vi "UIM Reg Notice wrapper.vi"(7 "b828NoticeDn":i32[](array[numeric])=[0, 0, 0, 0, 0, 0, 0, 0], 8 "error in (no error)":errorcluster caption="错误输入（无错误）", 9 "b828NoticeUp":i32[](array[numeric])=[0, 0, 0, 0, 0, 0, 0, 0], 10 "bDrvNotice":i32, 11 "pDummyCanIDNoticeUser":cluster{"dwDevIndex":u32, "dwCanNodeId":u32}) -> (0 "error out":errorcluster caption="错误输出", 1 "b828NoticeUp out":i32[](array[numeric]), 2 "function return":u32, 3 "pDummyCanIDNoticeUser out":cluster{"dwDevIndex":u32, "dwCanNodeId":u32}, 5 "b828NoticeDn out":i32[](array[numeric]))   [LabVIEW 2016, in "UISimCanFunc_wrapper.lvlib"]
doc: "_declspec (dllexport) DWORD UIMRegNotice_wrapper(P_DUMMY_CANIDNotice pDummyCanIDNoticeUser,\n BOOL bDrvNotice[NoticeSum], BOOL b828NoticeUp[8], BOOL b828NoticeDn[8]);"
uses:
  <userlib>/UISimCanFunc_wrapper/UISimCanFunc_wrapper.lvlib
  <userlib>/UISimCanFunc_wrapper/UISimCanFunc_wrapper.dll
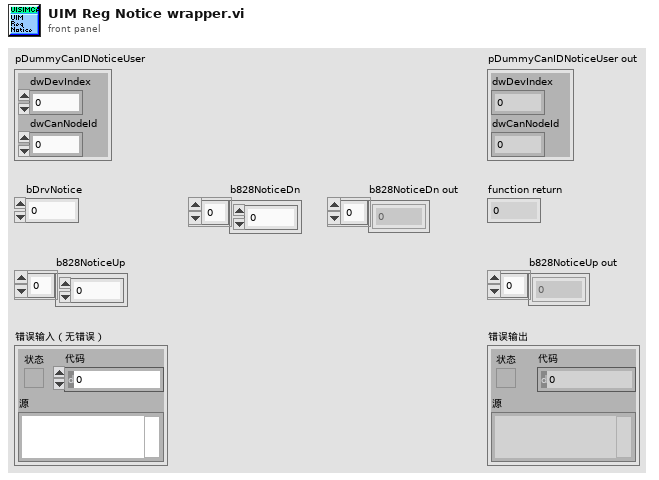
[diagram p1: front panel]
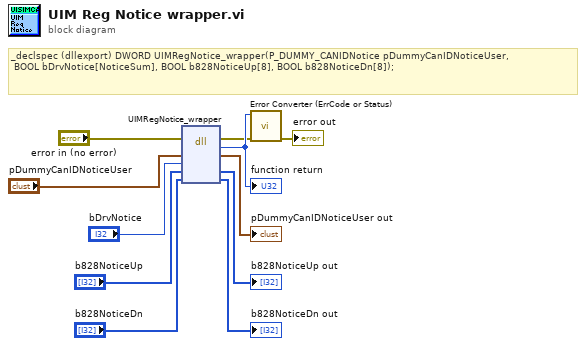
[diagram p0: block diagram]
diagram:
  # "_declspec (dllexport) DWORD UIMRegNotice_wrapper(P_DUMMY_CANIDNotice pDummyCanIDNoticeUser,\n\tBOOL bDrvNotice[NoticeSum], BOOL b828NoticeUp[8], BOOL b828NoticeDn[8]);"
  n1 = dll-call lib="C:/Program Files (x86)/National Instruments/LabVIEW 2016/user.lib/UISimCanFunc_wrapper/UISimCanFunc_wrapper.*" fn="UIMRegNotice_wrapper"(error in="error in (no error)", "pDummyCanIDNoticeUser"="pDummyCanIDNoticeUser", "bDrvNotice"="bDrvNotice", "b828NoticeUp"="b828NoticeUp", "b828NoticeDn"="b828NoticeDn") -> (error out=w2:errorcluster, w11:u32, "pDummyCanIDNoticeUser"=→"pDummyCanIDNoticeUser out":cluster{"dwDevIndex":u32, "dwCanNodeId":u32}, "b828NoticeUp"=→"b828NoticeUp out":i32[], "b828NoticeDn"=→"b828NoticeDn out":i32[])  [unwired: 3 in, 1 out]
  "function return" <- w11
  n2 = call <userlib>:"Error Converter (ErrCode or Status).vi"("error in (no error)"=w2, "error code"=w11) -> ("error out"=→"error out":errorcluster)  [unwired: 9 in]
